vi "GetOwner.vi"(8 "error in (no error)":errorcluster, 11 "SMO in":refnum<class "SMO.lvclass">) -> (0 "error out":errorcluster, 1 "found":bool, 2 "Owner":refnum<class "Attribute.Owner.lvclass">, 3 "SMO out":refnum<class "SMO.lvclass">)   [LabVIEW 2013, in "SMO.lvclass"]
uses:
  SMO.lvclass
  Support/Attribute.Owner/Attribute.Owner.lvclass
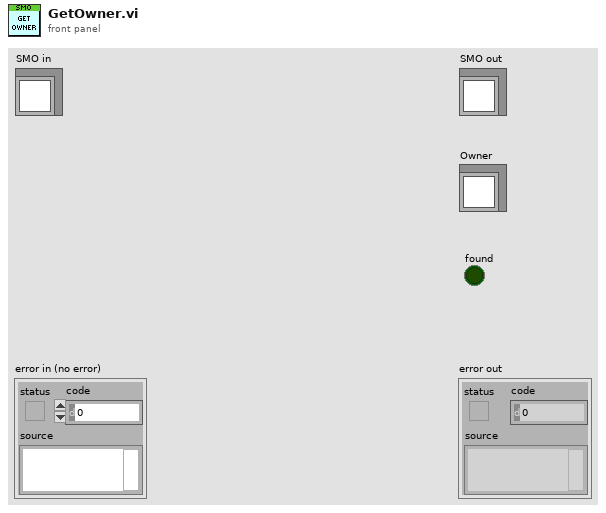
[diagram p1: front panel]
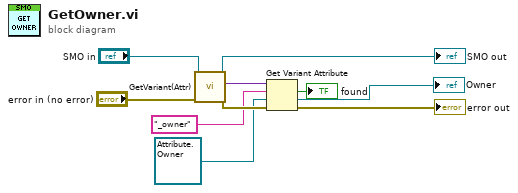
[diagram p0: block diagram]
diagram:
  n1 = call "GetVariant(Attr).vi"("error in (no error)"="error in (no error)", "SMO in"="SMO in") -> ("error out"=w9:errorcluster, "[Attributes]"=w10:variant, "SMO out"=→"SMO out":refnum<class "SMO.lvclass">)  [unwired: 7 in]
  n2 = Get Variant Attribute(Variant=w10, name="_owner", default value (empty Variant)=refnum<class "Attribute.Owner.lvclass"> refnum ("Attribute.Owner.lvclass"), error in=w9) -> (found=→"found":bool, value=→"Owner":refnum<class "Attribute.Owner.lvclass">, error out=→"error out":errorcluster)  [unwired: 1 out]
